vi "Get selected items.vi"(8 "error in (no error)":errorcluster, 11 "Pool":T1[](array[typedef])=[{"index"=0, "state"=enum."unused"}, {"index"=1, "state"=enum."unused"}, {"index"=2, "state"=enum."unused"}, {"index"=3, "state"=enum."unused"}, {"index"=4, "state"=enum."unused"}, {"index"=5, "state"=enum."unused"}]) -> (0 "error out":errorcluster, 1 "no. of selected items":i32, 2 "Selected indexes":i32[](array[numeric]), 3 "Selected items":T1[](array[typedef]))   [LabVIEW 2021, in "Numeric Utilities.lvlib"]
uses:
  Numeric Utilities.lvlib
  cluster-touched index.ctl
  index state enum.ctl
panel:
  # "Development\ncontrols/indicators useful for development and testing, but which are not outputs of the VI"
  # "Input\nInputs to the VI"
  # "Output\nOutputs of the VI"
  # "Description\n\nBlank VI with error handling case. \n\nSummarize the use of this VI in this space."
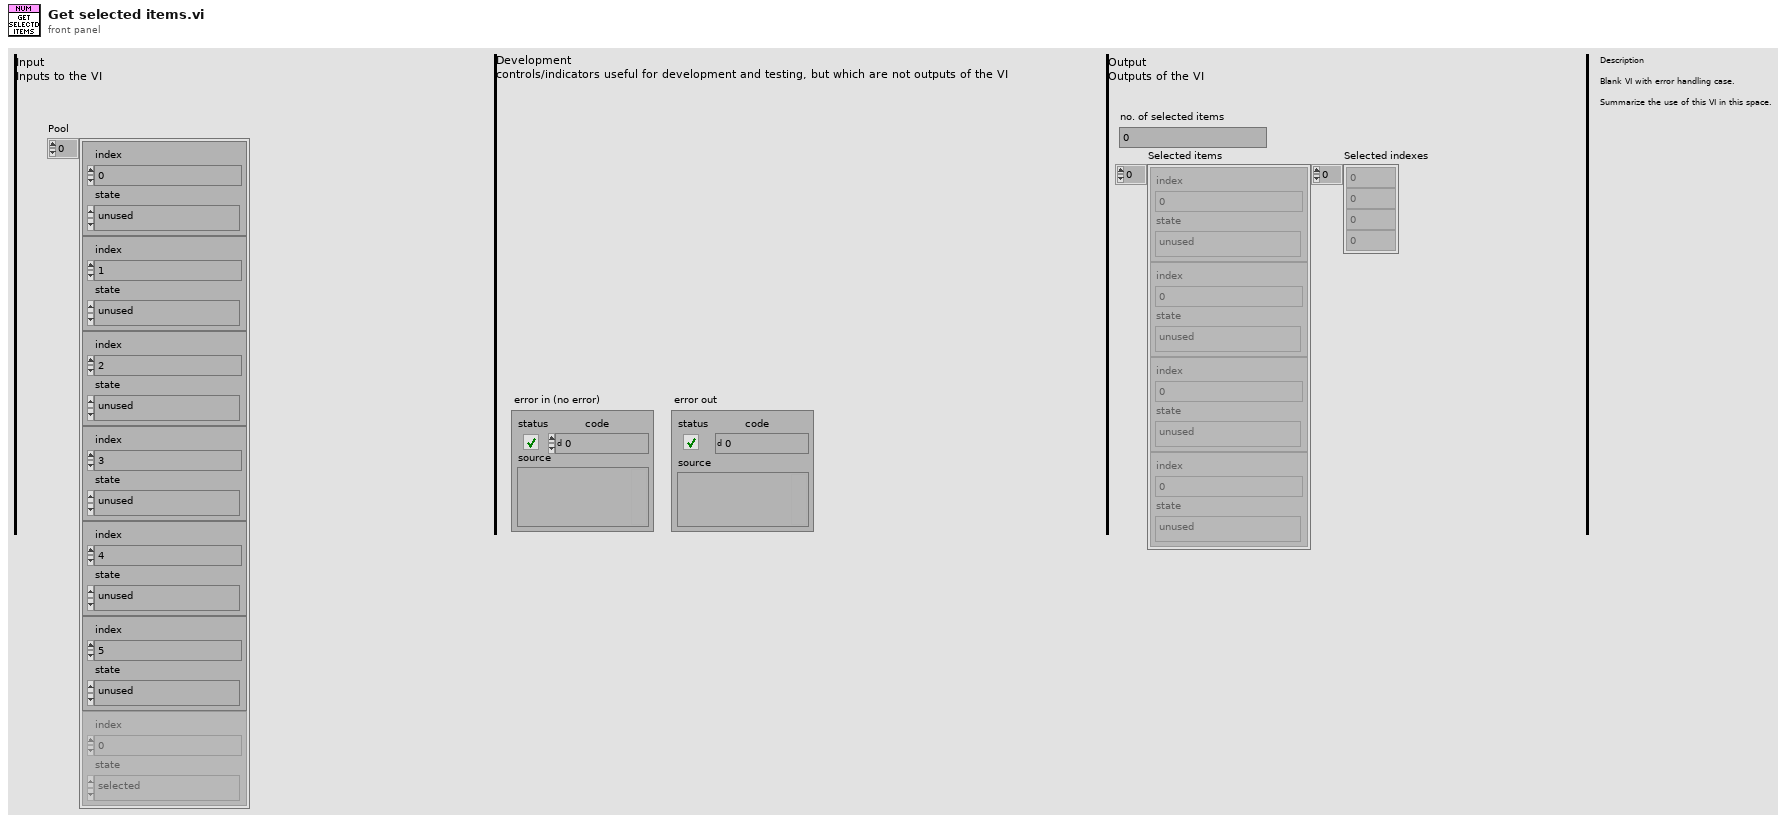
[diagram p1: front panel]
types:
  T1 = typedef "Numeric Utilities.lvlib/cluster-touched index.ctl" = cluster{"index":i32, "state":T2}
  T2 = typedef "Numeric Utilities.lvlib/index state enum.ctl" = enum16{"unused", "selected", "exhausted"}
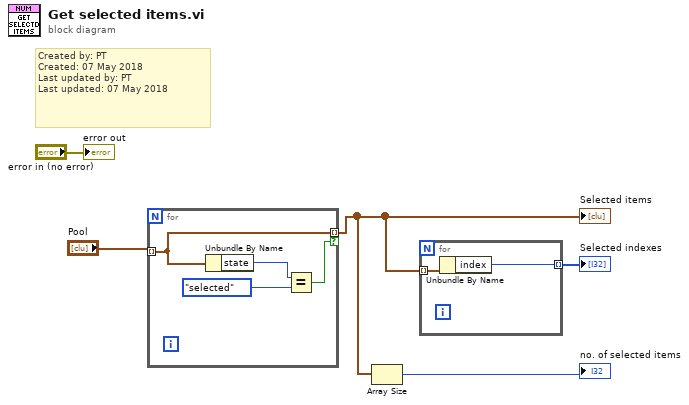
[diagram p0: block diagram]
diagram:
  # "Created by: PT\nCreated: 07 May 2018\nLast updated by: PT\nLast updated: 07 May 2018"
  n1 = for {
    tunnel: "Pool" -> [w7] mode=indexing
    tunnel: [w7] -> w2 mode=indexing if=w6
    n2 = Unbundle By Name(w7) -> ("state"=w9:T2)
    n3 = Equal?(x=w9, y=index_state_enum."selected") -> (x = y?=w6:bool)
  }
  "Selected items" <- w2
  n4 = Array Size(array=w2) -> (size(s)=→"no. of selected items":i32)
  n5 = for {
    tunnel: w2 -> [w11] mode=indexing
    tunnel: [w10] -> w1 mode=indexing
    n6 = Unbundle By Name(w11) -> ("index"=w10:i32)
  }
  "Selected indexes" <- w1
  "error out" <- "error in (no error)"
